vi "01-ConversaoCelsiusParaFahrenheit.vi"() -> ()   [LabVIEW 2014]
panel:
  out "Deg F":dbl
  in  "Deg C":dbl
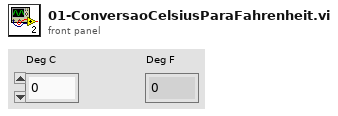
[diagram p1: front panel]
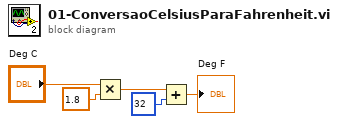
[diagram p0: block diagram]
diagram:
  n1 = Multiply(x="Deg C", y=1.8) -> (x*y=w3:dbl)
  n2 = Add(x=w3, y=32) -> (x+y=→"Deg F":dbl)
